vi "Convert to 32Bit Image.vi"(8 "error in (no error)":errorcluster, 11 "Image Data":T1) -> (0 "error out":errorcluster, 3 "32Bit Image Data Out":T1)   [LabVIEW 2019]
doc: "This VI will convert a set of <B>Image Data</B> into another set of <B>32Bit Image Data Out</B>. The image output will be the same as the input, with the addition that alpha layer information will have been set to solid for all pixels in the image.\n\n-----\nBrian Hoover (hooovahh)"
uses:
  <vilib>/picture/picture.llb/imagedata.ctl
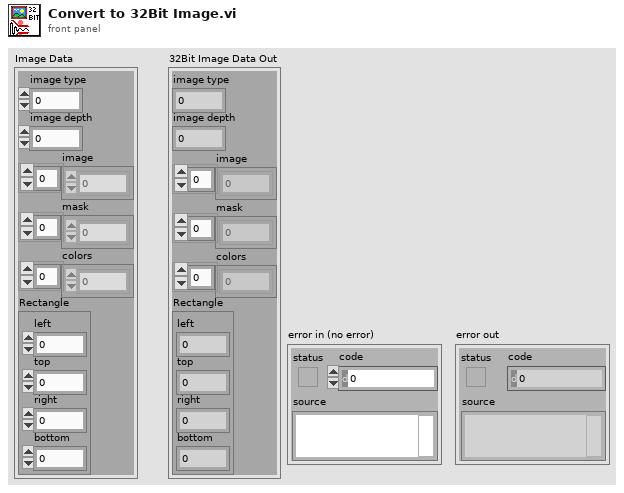
[diagram p1: front panel]
types:
  T1 = typedef "imagedata.ctl" = cluster{"image type":i32, "image depth":i32, "image":u8[], "mask":u8[], "colors":u32[], "Rectangle":cluster{"left":i16, "top":i16, "right":i16, "bottom":i16}}
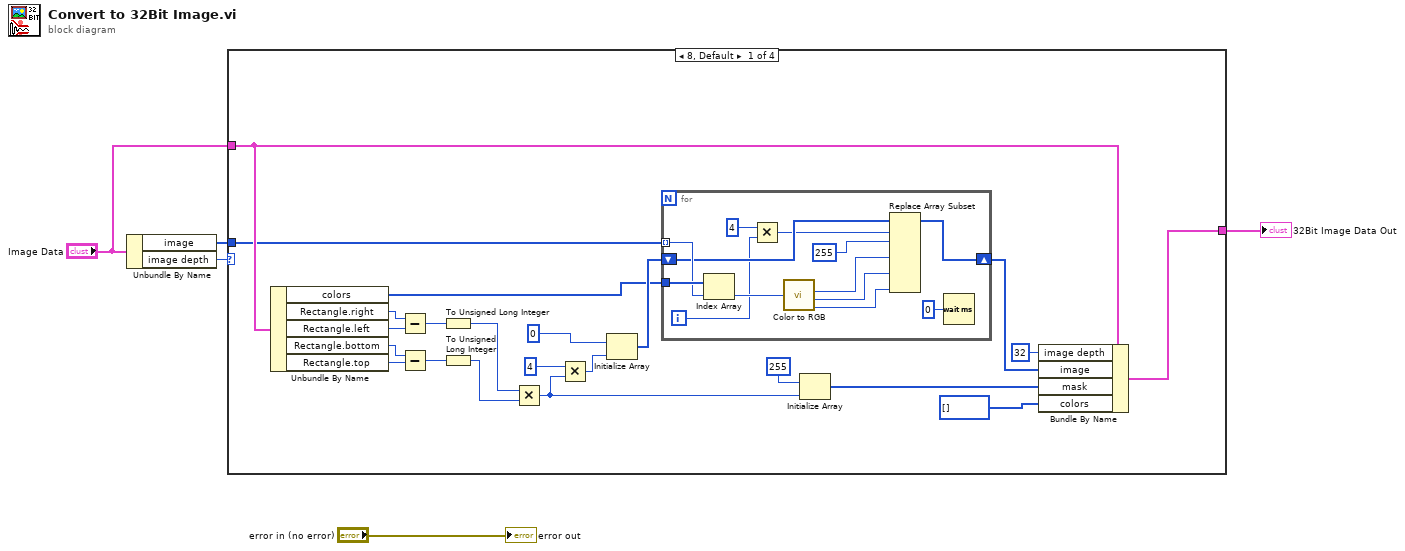
[diagram p0: block diagram]
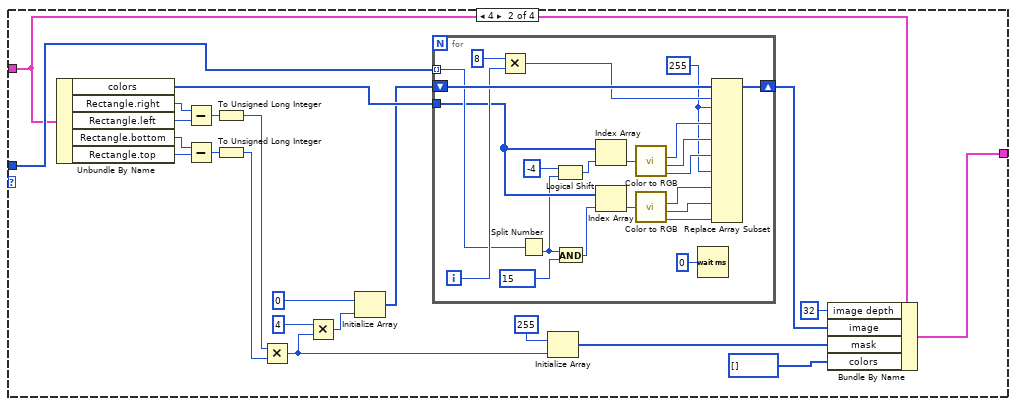
[diagram p2: hidden frame]
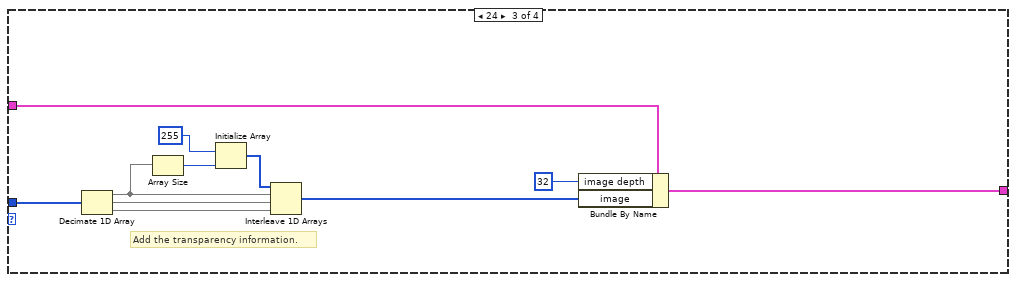
[diagram p3: hidden frame]
diagram:
  n1 = Unbundle By Name("Image Data") -> ("image"=w5:u8[], "image depth"=w2:i32)
  n2 = case shown="8, Default" w2 {
    tunnel: w5 -> [w7 w43 w95 _]
    tunnel: [w6 w41 w94 w96] -> w4
    tunnel: "Image Data" -> [w8 w42 w93 w96]
    frame 8, Default {
      n3 = Unbundle By Name(w8) -> ("colors"=w9:u32[], "Rectangle.right"=w20:i16, "Rectangle.left"=w21:i16, "Rectangle.bottom"=w22:i16, "Rectangle.top"=w23:i16)
      n4 = Subtract(x=w20, y=w21) -> (x-y=w25:i16)
      n5 = Subtract(x=w22, y=w23) -> (x-y=w24:i16)
      n6 = To Unsigned Long Integer(number=w25) -> (unsigned 32bit integer=w27:u32)
      n7 = To Unsigned Long Integer(number=w24) -> (unsigned 32bit integer=w26:u32)
      n8 = Multiply(x=w27, y=w26) -> (x*y=w19:u32)
      n9 = Multiply(x=u32 4, y=w19) -> (x*y=w16:u32)
      n10 = Initialize Array(u8 0, w16) -> (w18:u8[])
      n11 = for {
        tunnel: w7 -> [w39] mode=indexing
        tunnel: w9 -> [w40]
        shift-right: [w36] -> w10
        shift-left: w18 -> [w37]
        i -> [w35]
        n12 = Index Array(array=w40, index=w39) -> (element=w38:u32)
        n13 = Multiply(x=4, y=w35) -> (x*y=w33:i32)
        n14 = call <vilib>:"Color to RGB.vi"("Color"=w38) -> ("R"=w31:u8, "G"=w30:u8, "B"=w29:u8)  [unwired: 1 out]
        n15 = Replace Array Subset(array=w37, new element #1=u8 255 ("B"), index #1=w33, new element #2=w31, new element #3=w30, new element #4=w29) -> (w36:u8[])  [unwired: 3 in]
        n16 = Wait (ms)(milliseconds to wait=u32 0) -> ()  [unwired: 1 out]
      }
      n17 = Initialize Array(u8 255, w19) -> (w14:u8[])
      n18 = Bundle By Name(cluster=w8, "image depth"=32, "image"=w10, "mask"=w14, "colors"=u32[] []) -> (w6:T1)
    }
    frame 4 {
      n19 = Unbundle By Name(w42) -> ("colors"=w62:u32[], "Rectangle.right"=w51:i16, "Rectangle.left"=w50:i16, "Rectangle.bottom"=w49:i16, "Rectangle.top"=w48:i16)
      n20 = Subtract(x=w51, y=w50) -> (x-y=w46:i16)
      n21 = Subtract(x=w49, y=w48) -> (x-y=w47:i16)
      n22 = To Unsigned Long Integer(number=w46) -> (unsigned 32bit integer=w44:u32)
      n23 = To Unsigned Long Integer(number=w47) -> (unsigned 32bit integer=w45:u32)
      n24 = Multiply(x=w44, y=w45) -> (x*y=w52:u32)
      n25 = Multiply(x=u32 4, y=w52) -> (x*y=w55:u32)
      n26 = Initialize Array(u8 0, w55) -> (w53:u8[])
      n27 = for {
        tunnel: w43 -> [w74] mode=indexing
        tunnel: w62 -> [w72]
        shift-right: [w82] -> w61
        shift-left: w53 -> [w83]
        i -> [w81]
        w71 = u8 255 ("B")
        n28 = Multiply(x=8, y=w81) -> (x*y=w79:i32)
        n29 = Split Number(x=w74) -> (lo(x)=w64:u8)  [unwired: 1 out]
        n30 = Logical Shift(y=-4 ("x"), x=w64) -> (x << y=w65:u8)
        n31 = And(x=w64, y=u8 15) -> (x .and. y?=w66:u8)
        n32 = Index Array(array=w72, index=w65) -> (element=w84:u32)
        n33 = Index Array(array=w72, index=w66) -> (element=w73:u32)
        n34 = call <vilib>:"Color to RGB.vi"("Color"=w84) -> ("R"=w78:u8, "G"=w77:u8, "B"=w76:u8)  [unwired: 1 out]
        n35 = call <vilib>:"Color to RGB.vi"("Color"=w73) -> ("R"=w70:u8, "G"=w69:u8, "B"=w68:u8)  [unwired: 1 out]
        n36 = Wait (ms)(milliseconds to wait=u32 0) -> ()  [unwired: 1 out]
        n37 = Replace Array Subset(array=w83, new element #1=w71, index #1=w79, new element #2=w78, new element #3=w77, new element #4=w76, new element #5=w71, new element #6=w70, new element #7=w69, new element #8=w68) -> (w82:u8[])  [unwired: 7 in]
      }
      n38 = Initialize Array(u8 255, w52) -> (w57:u8[])
      n39 = Bundle By Name(cluster=w42, "image depth"=32, "image"=w61, "mask"=w57, "colors"=u32[] []) -> (w41:T1)
    }
    frame 24 {
      # "Add the transparency information."
      n40 = Decimate 1D Array(w95) -> (w88:u8[], w89:u8[], w90:u8[])
      n41 = Array Size(array=w88) -> (size(s)=w87:i32)
      n42 = Initialize Array(u8 255, w87) -> (w85:u8[])
      n43 = Interleave 1D Arrays(w85, w88, w89, w90) -> (w91:u8[])
      n44 = Bundle By Name(cluster=w93, "image depth"=32, "image"=w91) -> (w94:T1)
    }
    frame 32 {
    }
  }
  "32Bit Image Data Out" <- w4
  "error out" <- "error in (no error)"
